vi "Fighter.vi"(8 "error in (no error)":errorcluster, 10 "Map":i32[](array[numeric]), 11 "Fighter In":refnum<class "Cross.lvclass">) -> (0 "error out":errorcluster, 1 "Direction":T1, 2 "Action":T2, 3 "Fighter Out":refnum<class "Cross.lvclass">, 4 "Replicated Class":refnum<class "Cross.lvclass">)   [LabVIEW 2015, in "Cross.lvclass"]
uses:
  Cross.lvclass
  Type Defs/Action Enum.ctl
  Type Defs/Direction Enum.ctl
  Cross.lvclass/Cross.ctl
  Type Defs/SB Type Defs.lvlib
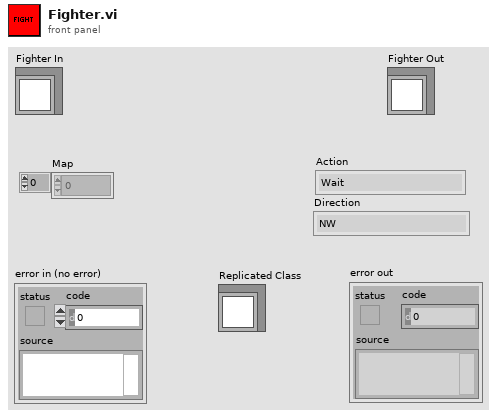
[diagram p1: front panel]
types:
  T1 = typedef "SB Type Defs.lvlib/Direction Enum.ctl" = enum16{"NW", "N", "NE", "E", "SE", "S", "SW", "W"}
  T2 = typedef "SB Type Defs.lvlib/Action Enum.ctl" = enum16{"Wait", "Move", "Attack", "Replicate"}
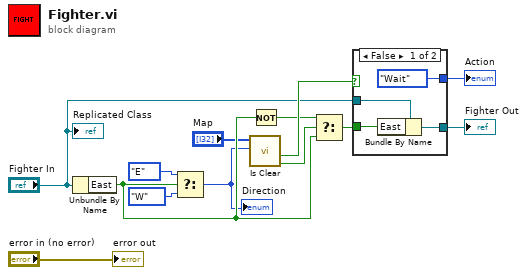
[diagram p0: block diagram]
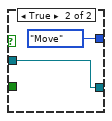
[diagram p2: hidden frame]
diagram:
  n1 = Unbundle By Name("Fighter In") -> ("East"=w8:bool)
  n2 = Select(t=Direction_Enum."E" ("Direction"), s=w8, f=Direction_Enum."W" ("Direction")) -> (s? t:f=w1:T1)
  "Direction" <- w1
  n3 = call "Is Clear.vi"("Direction"=w1, "Maze"="Map") -> ("Blocked?"=w7:bool, "Can Move?"=w10:bool)  [unwired: 6 in, 2 out]
  n4 = Not(x=w8) -> (.not. x?=w6:bool)
  n5 = Select(t=w6, s=w7, f=w8) -> (s? t:f=w9:bool)
  n6 = case shown="False" w10 {
    tunnel: [Action_Enum."Wait" ("Action") Action_Enum."Move" ("Action")] -> w2
    tunnel: "Fighter In" -> [w16 w18]
    tunnel: w9 -> [w14 _]
    tunnel: [w15 w18] -> w3
    frame False {
      n7 = Bundle By Name(cluster=w16, "East"=w14) -> (w15:refnum<class "Cross.lvclass">)
    }
    frame True {
    }
  }
  "Action" <- w2
  "Fighter Out" <- w3
  "error out" <- "error in (no error)"
  "Replicated Class" <- "Fighter In"
